vi "PPR_DRIVE_GLOBALS.vi"() -> ()   [LabVIEW 2019]
uses:
  <vilib>/Rock Robotics/WPI/ThirdParty/JAS_Junk/TrajLib/TypeDef/DIFF_DRIVE_KINEMATICS.ctl
  <vilib>/Rock Robotics/WPI/ThirdParty/JAS_Junk/TrajLib/Trajectory_Library.lvlib
panel:
  out "Right Wheel Speed Err M/S":dbl format="%17.2f"
  out "Left Wheel Speed Err M/S":dbl format="%17.2f"
  out "Right Wheel Limited Speed Dmd M/S":dbl format="%17.2f"
  out "Left Wheel Limited Speed Dmd M/S":dbl format="%17.2f"
  out "Right Wheel Speed Dmd M/s":dbl format="%17.2f"
  out "Left Wheel Speed Dmd M/S":dbl format="%17.2f"
  out "Right Wheel Motor Out":dbl format="%17.3f"
  out "Left Wheel Motor Out":dbl format="%17.3f"
  out "Right Wheel Speed M/S":dbl format="%17.2f"
  out "Left Wheel Speed M/S":dbl format="%17.2f"
  out "Right Wheel Dist M":dbl format="%17.2f"
  out "Left Wheel Dist M":dbl format="%17.2f"
  out "Closed Loop Ctrl":bool
  out "Orientation_Angle_Demand_Radians":dbl format="%17.2f"
  out "DIFF_DRIVE_KINEMATICS":T1 {"TrackWidth_Meters" format="%20.4f"}
  out "GyroHeading_Radians":dbl format="%17.2f"
  out "Orientation Correct CO":dbl format="%17.3f"
  out "Orientation Angle Error_Rad":dbl format="%17.3f"
  # "Orientation Correction data"
  # "Sensor Readings"
  # "Actuator Outputs"
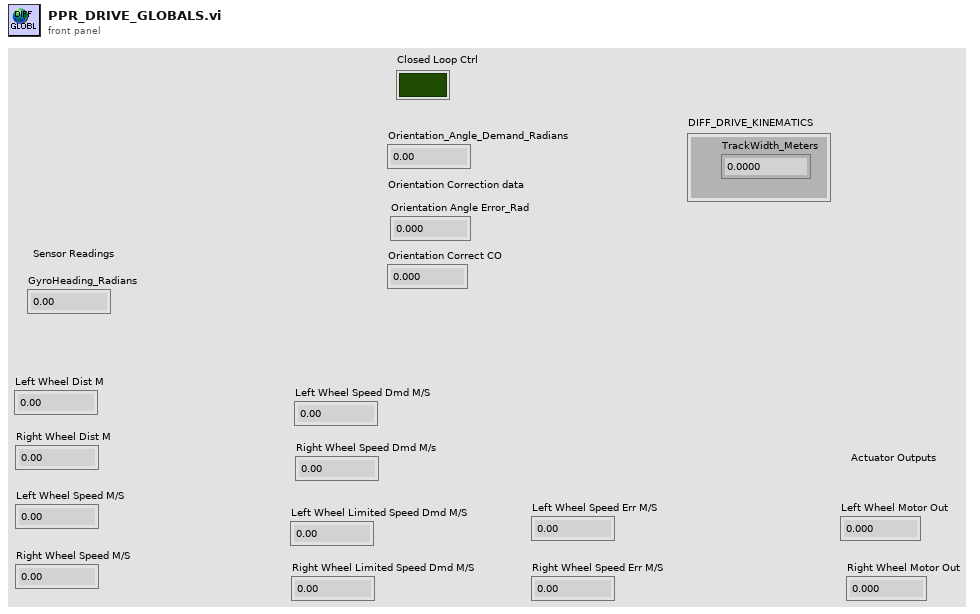
[diagram p1: front panel]
types:
  T1 = typedef "Trajectory_Library.lvlib/DIFF_DRIVE_KINEMATICS.ctl" = cluster{"TrackWidth_Meters":dbl}
diagram:
